vi "osie na grafie.vi"(8 "Y axis rotation":i32, 9 "X axis rotation":i32, 10 "X axis":i32, 11 "Y axis":i32) -> (0 "graph 2":cluster{i32[], i32[]}[](graph))   [LabVIEW 2015]
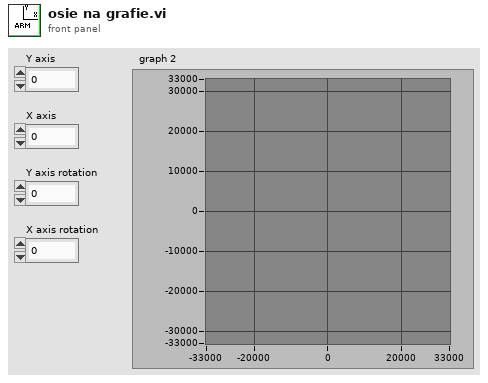
[diagram p1: front panel]
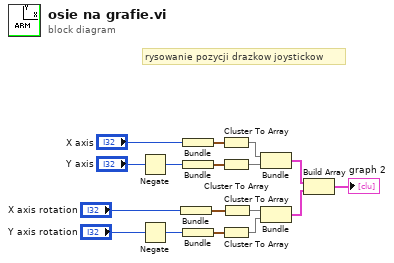
[diagram p0: block diagram]
diagram:
  # "rysowanie pozycji drazkow joystickow"
  n1 = Negate(x="Y axis") -> (-x=w4:i32)
  n2 = Negate(x="Y axis rotation") -> (-x=w9:i32)
  n3 = Bundle("X axis rotation"="X axis rotation") -> (w10:cluster{"X axis rotation":i32})  [unwired: 1 in]
  n4 = Bundle("X axis"="X axis") -> (w3:cluster{"X axis":i32})  [unwired: 1 in]
  n5 = Bundle(w4) -> (w5:cluster{i32})  [unwired: 1 in]
  n6 = Bundle(w9) -> (w8:cluster{i32})  [unwired: 1 in]
  n7 = Cluster To Array(cluster=w3) -> (array=w2:i32[])
  n8 = Cluster To Array(cluster=w5) -> (array=w1:i32[])
  n9 = Cluster To Array(cluster=w8) -> (array=w12:i32[])
  n10 = Cluster To Array(cluster=w10) -> (array=w11:i32[])
  n11 = Bundle(w2, w1) -> (w16:cluster{i32[], i32[]})  [unwired: 1 in]
  n12 = Bundle(w11, w12) -> (w15:cluster{i32[], i32[]})  [unwired: 1 in]
  n13 = Build Array(w16, w15) -> (→"graph 2":cluster{i32[], i32[]}[])
